vi "Find.vi"(4 "limitInteger":i32, 6 "sortString":string, 8 "error in (no error)":errorcluster, 9 "filterString":string, 10 "selectionString":string, 11 "MongoDB-Collection in":refnum<class "MongoDB-Collection.lvclass">) -> (0 "error out":errorcluster, 2 "Find":string[](array[string]), 3 "MongoDB-Collection out":refnum<class "MongoDB-Collection.lvclass">)   [LabVIEW 2016, in "MongoDB-Collection.lvlib" / "MongoDB-Collection.lvclass"]
uses:
  MongoDB-Collection.lvclass
  D:/Users/blume/Desktop/LV/MongoDB-Driver/MLV DLLs/MongoLabVIEW.dll
  LV/MongoDB-Driver/MLV DLLs/MongoLabVIEW.dll
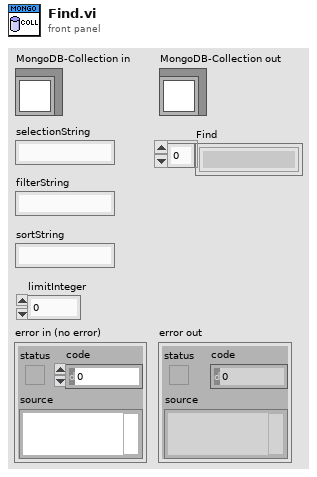
[diagram p1: front panel]
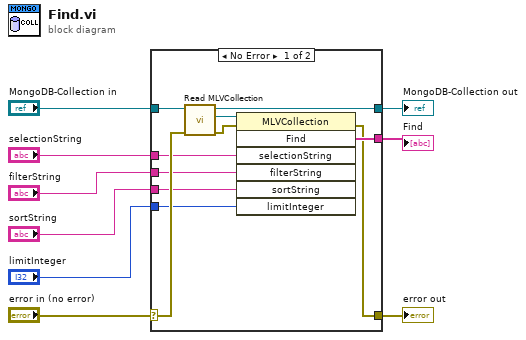
[diagram p0: block diagram]
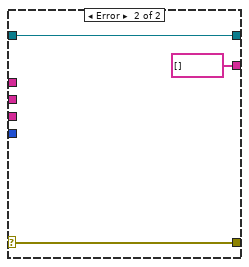
[diagram p2: hidden frame]
diagram:
  n1 = case shown="No Error" "error in (no error)" {
    selector: "error in (no error)" -> [w19 w23]
    tunnel: [w10 w23] -> w8
    tunnel: [w18 w22] -> w6
    tunnel: "MongoDB-Collection in" -> [w20 w22]
    tunnel: "selectionString" -> [w15 _]
    tunnel: "filterString" -> [w14 _]
    tunnel: "sortString" -> [w13 _]
    tunnel: "limitInteger" -> [w12 _]
    tunnel: [w11 string[] [] ("Find")] -> w1
    frame No Error {
      n2 = call "Read MLVCollection.vi"("error in (no error)"=w19, "MongoDB-Collection in"=w20) -> ("error out"=w16:errorcluster, "MLVCollection"=w17:refnum<k24>, "MongoDB-Collection out"=w18:refnum<class "MongoDB-Collection.lvclass">)  [unwired: 7 in]
      n3 = invoke class="MLVCollection" method="Find"(reference=w17, error in=w16, "selectionString"=w15, "filterString"=w14, "sortString"=w13, "limitInteger"=w12) -> (error out=w10:errorcluster, "Find"=w11:string[])  [unwired: 1 in, 5 out]
    }
    frame Error {
    }
  }
  "error out" <- w8
  "MongoDB-Collection out" <- w6
  "Find" <- w1
